vi "4Linea2.vi"(11 "array":string[][](array[string])) -> (3 "x .or. y?":bool)   [LabVIEW 2020]
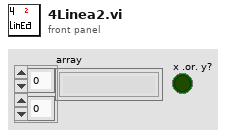
[diagram p1: front panel]
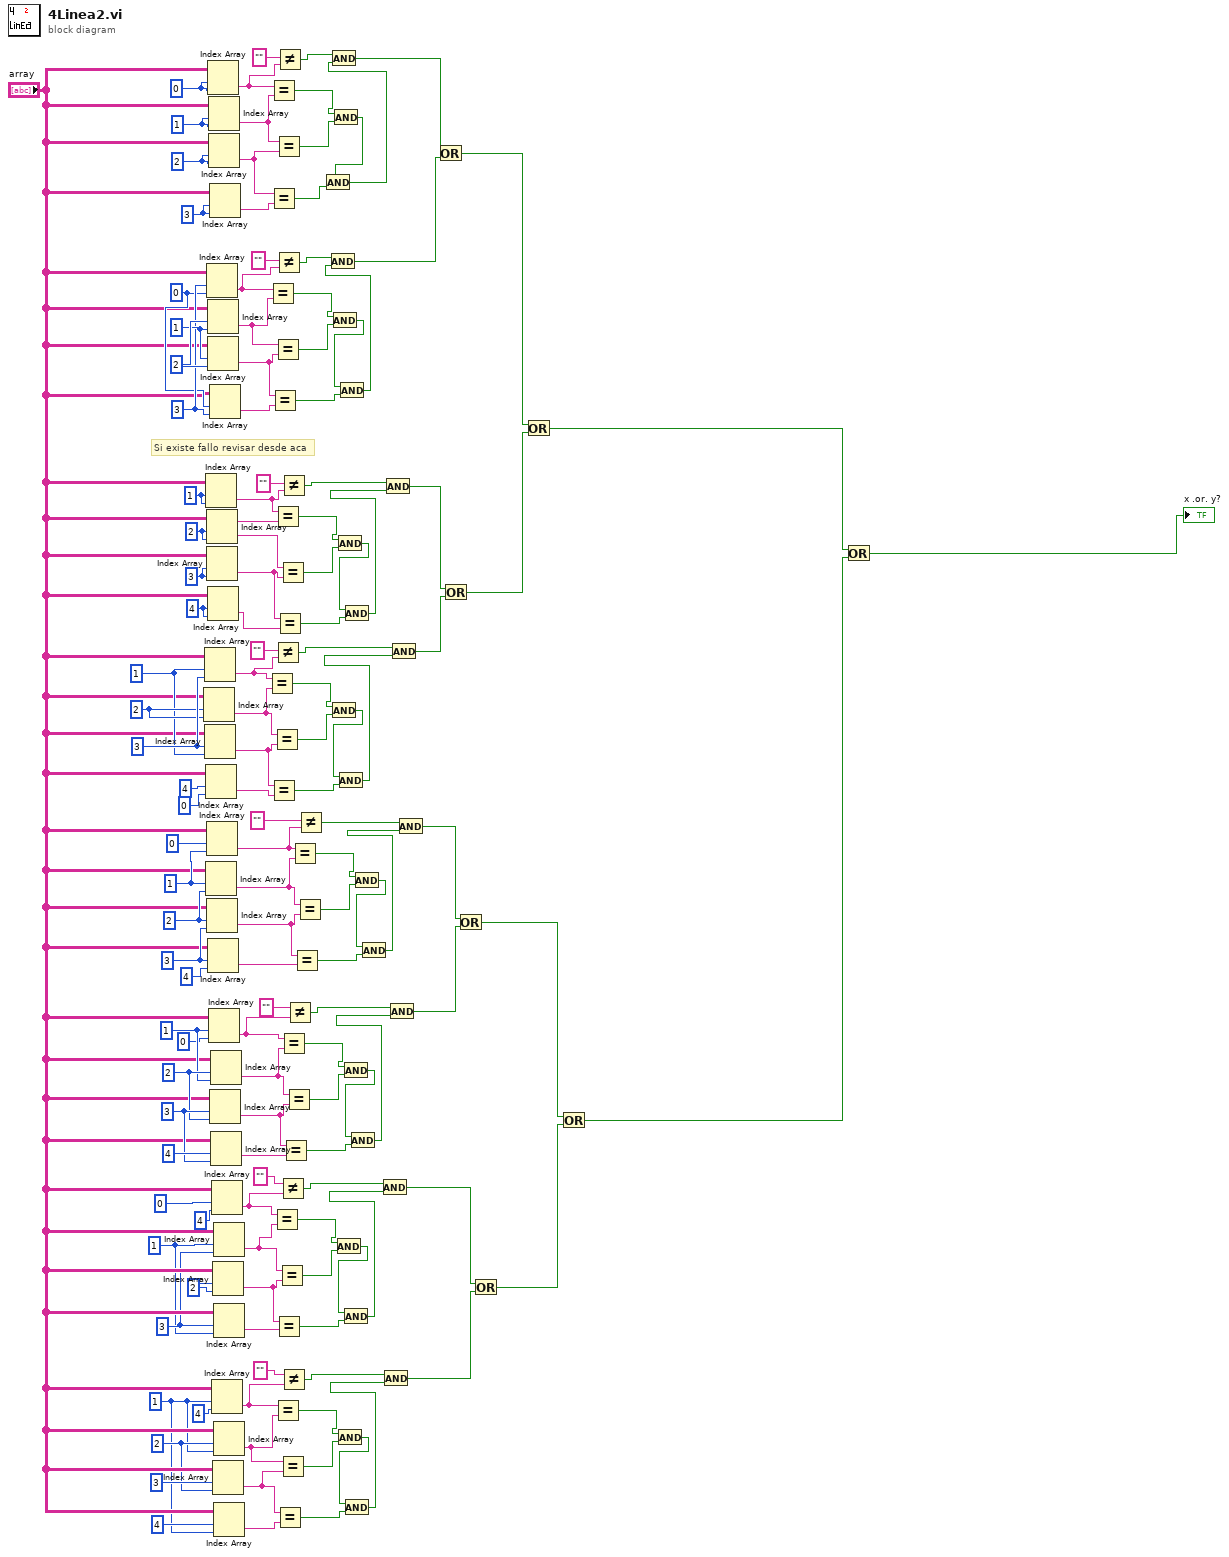
[diagram p0: block diagram]
diagram:
  w23 = 2 ("index (row)")
  w22 = 1 ("index (row)")
  w39 = 3 ("index (row)")
  w38 = 2 ("index (row)")
  w37 = 1 ("index (row)")
  w59 = 3 ("index (row)")
  w58 = 2 ("index (row)")
  w57 = 1 ("index (row)")
  w73 = 3 ("index (row)")
  w74 = 2 ("index (row)")
  w75 = 1 ("index (row)")
  w86 = 3 ("index (row)")
  w85 = 2 ("index (row)")
  w84 = 1 ("index (row)")
  w106 = 4 ("index (row)")
  w107 = 3 ("disabled index (col)")
  w108 = 2 ("index (row)")
  w109 = 1 ("index (row)")
  w116 = 3
  w124 = 3 ("index (col)")
  w118 = 2
  w117 = 1
  w115 = 0
  w139 = 2
  w140 = 1
  w141 = 0
  # "Si existe fallo revisar desde aca"
  n1 = Index Array(array="array", index (row)=w85, index (col)=w85) -> (element=w81:string)
  n2 = Index Array(array="array", index (row)=w84, index (col)=w86) -> (element=w82:string)
  n3 = Index Array(array="array", index (row)=w86, index (col)=w84) -> (element=w80:string)
  n4 = Index Array(array="array", index (row)=w109, index (col)=w109) -> (element=w91:string)
  n5 = Index Array(array="array", index (row)=4, index (col)=0 ("disabled index (col)")) -> (element=w79:string)
  n6 = Index Array(array="array", index (row)=w75, index (col)=w74) -> (element=w64:string)
  n7 = Index Array(array="array", index (row)=w116, index (col)=w115) -> (element=w127:string)
  n8 = Index Array(array="array", index (row)=w108, index (col)=w108) -> (element=w90:string)
  n9 = Index Array(array="array", index (row)=w107, index (col)=w107) -> (element=w89:string)
  n10 = Index Array(array="array", index (row)=0, index (col)=w75) -> (element=w61:string)
  n11 = Index Array(array="array", index (row)=w74, index (col)=w73) -> (element=w62:string)
  n12 = Index Array(array="array", index (row)=w141, index (col)=w141) -> (element=w133:string)
  n13 = Index Array(array="array", index (row)=w118, index (col)=w117) -> (element=w128:string)
  n14 = Index Array(array="array", index (row)=w117, index (col)=w118) -> (element=w113:string)
  n15 = Index Array(array="array", index (row)=w106, index (col)=w106) -> (element=w88:string)
  n16 = Index Array(array="array", index (row)=w73, index (col)=4 ("disabled index (col)")) -> (element=w63:string)
  n17 = Index Array(array="array", index (row)=w140, index (col)=w140) -> (element=w138:string)
  n18 = Index Array(array="array", index (row)=w139, index (col)=w139) -> (element=w122:string)
  n19 = Index Array(array="array", index (row)=w57, index (col)=0 ("disabled index (col)")) -> (element=w48:string)
  n20 = Index Array(array="array", index (row)=w124, index (col)=w124) -> (element=w123:string)
  n21 = Index Array(array="array", index (row)=w115, index (col)=w116) -> (element=w114:string)
  n22 = Index Array(array="array", index (row)=w59, index (col)=w58) -> (element=w46:string)
  n23 = Index Array(array="array", index (row)=w58, index (col)=w57) -> (element=w47:string)
  n24 = Index Array(array="array", index (row)=4, index (col)=w59) -> (element=w45:string)
  n25 = Index Array(array="array", index (row)=0, index (col)=4 ("disabled index (col)")) -> (element=w30:string)
  n26 = Index Array(array="array", index (row)=w22, index (col)=4 ("disabled index (col)")) -> (element=w14:string)
  n27 = Index Array(array="array", index (row)=w38, index (col)=w38) -> (element=w28:string)
  n28 = Index Array(array="array", index (row)=3, index (col)=w23) -> (element=w12:string)
  n29 = Index Array(array="array", index (row)=w37, index (col)=w39) -> (element=w29:string)
  n30 = Index Array(array="array", index (row)=w39, index (col)=w37) -> (element=w27:string)
  n31 = Index Array(array="array", index (row)=w23, index (col)=w22) -> (element=w13:string)
  n32 = Index Array(array="array", index (row)=4, index (col)=w22) -> (element=w11:string)
  n33 = Equal?(x=w82, y=w81) -> (x = y?=w102:bool)
  n34 = Equal?(x=w127, y=w128) -> (x = y?=w129:bool)
  n35 = Equal?(x=w133, y=w138) -> (x = y?=w137:bool)
  n36 = Equal?(x=w122, y=w123) -> (x = y?=w121:bool)
  n37 = Equal?(x=w80, y=w79) -> (x = y?=w101:bool)
  n38 = Equal?(x=w113, y=w114) -> (x = y?=w112:bool)
  n39 = Equal?(x=w81, y=w80) -> (x = y?=w103:bool)
  n40 = Equal?(x=w30, y=w29) -> (x = y?=w34:bool)
  n41 = Equal?(x=w128, y=w113) -> (x = y?=w130:bool)
  n42 = Equal?(x=w91, y=w90) -> (x = y?=w95:bool)
  n43 = Not Equal?(x="", y=w82) -> (x != y?=w104:bool)
  n44 = Equal?(x=w14, y=w13) -> (x = y?=w18:bool)
  n45 = Equal?(x=w138, y=w122) -> (x = y?=w136:bool)
  n46 = Not Equal?(x="", y=w127) -> (x != y?=w131:bool)
  n47 = Equal?(x=w28, y=w27) -> (x = y?=w33:bool)
  n48 = Not Equal?(x="", y=w133) -> (x != y?=w135:bool)
  n49 = Equal?(x=w89, y=w88) -> (x = y?=w94:bool)
  n50 = Equal?(x=w12, y=w11) -> (x = y?=w17:bool)
  n51 = Equal?(x=w29, y=w28) -> (x = y?=w35:bool)
  n52 = Equal?(x=w90, y=w89) -> (x = y?=w96:bool)
  n53 = Not Equal?(x="", y=w30) -> (x != y?=w36:bool)
  n54 = Equal?(x=w13, y=w12) -> (x = y?=w19:bool)
  n55 = Not Equal?(x="", y=w91) -> (x != y?=w97:bool)
  n56 = Equal?(x=w48, y=w47) -> (x = y?=w53:bool)
  n57 = Not Equal?(x="", y=w14) -> (x != y?=w20:bool)
  n58 = Equal?(x=w46, y=w45) -> (x = y?=w52:bool)
  n59 = Equal?(x=w47, y=w46) -> (x = y?=w54:bool)
  n60 = Not Equal?(x="", y=w48) -> (x != y?=w55:bool)
  n61 = Equal?(x=w61, y=w64) -> (x = y?=w68:bool)
  n62 = Equal?(x=w62, y=w63) -> (x = y?=w67:bool)
  n63 = Equal?(x=w64, y=w62) -> (x = y?=w69:bool)
  n64 = Not Equal?(x="", y=w61) -> (x != y?=w70:bool)
  n65 = And(x=w102, y=w103) -> (x .and. y?=w100:bool)
  n66 = And(x=w129, y=w130) -> (x .and. y?=w111:bool)
  n67 = And(x=w137, y=w136) -> (x .and. y?=w120:bool)
  n68 = And(x=w120, y=w121) -> (x .and. y?=w119:bool)
  n69 = And(x=w135, y=w119) -> (x .and. y?=w126:bool)
  n70 = And(x=w34, y=w35) -> (x .and. y?=w32:bool)
  n71 = And(x=w95, y=w96) -> (x .and. y?=w93:bool)
  n72 = And(x=w18, y=w19) -> (x .and. y?=w16:bool)
  n73 = And(x=w100, y=w101) -> (x .and. y?=w99:bool)
  n74 = And(x=w111, y=w112) -> (x .and. y?=w110:bool)
  n75 = And(x=w131, y=w110) -> (x .and. y?=w125:bool)
  n76 = And(x=w53, y=w54) -> (x .and. y?=w51:bool)
  n77 = And(x=w32, y=w33) -> (x .and. y?=w31:bool)
  n78 = And(x=w93, y=w94) -> (x .and. y?=w92:bool)
  n79 = And(x=w16, y=w17) -> (x .and. y?=w15:bool)
  n80 = And(x=w51, y=w52) -> (x .and. y?=w50:bool)
  n81 = And(x=w68, y=w69) -> (x .and. y?=w66:bool)
  n82 = And(x=w66, y=w67) -> (x .and. y?=w65:bool)
  n83 = And(x=w36, y=w31) -> (x .and. y?=w9:bool)
  n84 = And(x=w20, y=w15) -> (x .and. y?=w8:bool)
  n85 = And(x=w97, y=w92) -> (x .and. y?=w78:bool)
  n86 = And(x=w55, y=w50) -> (x .and. y?=w43:bool)
  n87 = And(x=w104, y=w99) -> (x .and. y?=w77:bool)
  n88 = And(x=w70, y=w65) -> (x .and. y?=w44:bool)
  n89 = Or(x=w126, y=w125) -> (x .or. y?=w7:bool)
  n90 = Or(x=w78, y=w77) -> (x .or. y?=w6:bool)
  n91 = Or(x=w44, y=w43) -> (x .or. y?=w5:bool)
  n92 = Or(x=w9, y=w8) -> (x .or. y?=w4:bool)
  n93 = Or(x=w7, y=w6) -> (x .or. y?=w3:bool)
  n94 = Or(x=w5, y=w4) -> (x .or. y?=w2:bool)
  n95 = Or(x=w3, y=w2) -> (x .or. y?=→"x .or. y?":bool)
